vi "FABR-Plot Progress Bars.vi"(0 "Analysis":T1, 2 "Neural Ref":refnum<vi>, 7 "finished":bool, 11 "error in (no error)":errorcluster) -> (15 "error out":errorcluster)   [LabVIEW 2020]
uses:
  Typedefs/FABR-Analysis State.ctl
  Threshold Estimation VIs/ABR3-Threshold Estimation Result.ctl
panel:
  # "Freq X Level X Time"
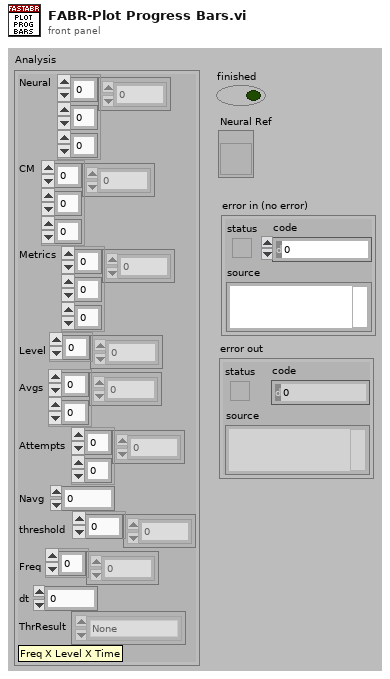
[diagram p1: front panel]
types:
  T1 = typedef "FABR-Analysis State.ctl" = cluster{"Neural":dbl[][][], "CM":dbl[][][], "Metrics":dbl[][][], "Level":dbl[], "Avgs":i32[][], "Attempts":i32[][], "Navg":i32, "threshold":dbl[], "Freq":dbl[], "dt":dbl, "ThrResult":T2[]}
  T2 = typedef "ABR3-Threshold Estimation Result.ctl" = enum16{"None", "Power", "Sigmoid", "Power (noisy)", "Suprathreshold", "Invalid"}
  T3 = typedef "LVRectTypeDef.ctl" = cluster{"Left":i16, "Top":i16, "Right":i16, "Bottom":i16}
  T4 = cluster{"Width":i16, "Style":enum32{"Solid", "Dash", "Dot", "DashDot", "DashDotDot"}}
  T5 = typedef "LVPoint32TypeDef.ctl" = cluster{"Horizontal":i32, "Vertical":i32}
  T6 = cluster{"Horizontal":i32, i32, "Horizontal":i32, i32}
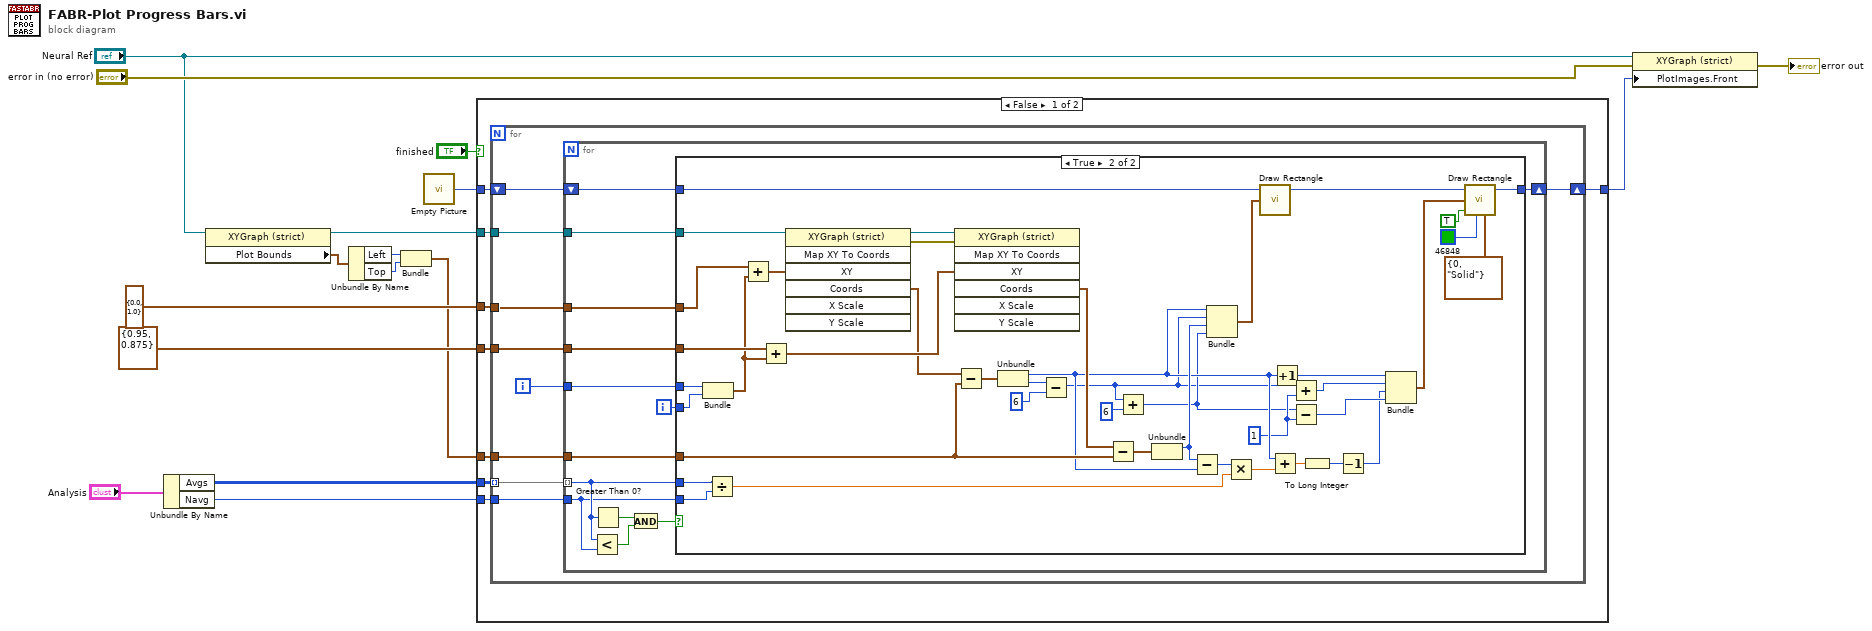
[diagram p0: block diagram]
diagram:
  n1 = Unbundle By Name("Analysis") -> ("Avgs"=w13:i32[][], "Navg"=w8:i32)
  n2 = property class="XYGraph (strict)"(reference="Neural Ref") -> (reference out=w7:refnum<vi>, "Plot Bounds"=w5:T3)  [unwired: 1 in, 1 out]
  n3 = Unbundle By Name(w5) -> ("Left"=w4:i16, "Top"=w3:i16)
  n4 = Bundle("Left"=w4, "Top"=w3) -> (w2:cluster{"Left":i16, "Top":i16})  [unwired: 1 in]
  n5 = call "Empty Picture"() -> ("empty picture"=w12:picture)
  n6 = case shown="False" "finished" {
    tunnel: w13 -> [w24 _]
    tunnel: w12 -> [w23 w90]
    tunnel: [w22 w90] -> w11
    tunnel: cluster{"X":dbl, "Y":dbl} {"X"=0.0, "Y"=1.0} ("XY") -> [w21 _]
    tunnel: cluster{"X":dbl, "Y":dbl} {"X"=0.95, "Y"=0.875} ("XY") -> [w20 _]
    tunnel: w8 -> [w19 _]
    tunnel: w7 -> [w18 _]
    tunnel: w2 -> [w17 _]
    frame False {
      n7 = for {
        tunnel: w24 -> [w28] mode=indexing
        shift-right: [w32] -> w22
        shift-left: w23 -> [w33]
        tunnel: w21 -> [w31]
        tunnel: w18 -> [w29]
        tunnel: w20 -> [w27]
        tunnel: w19 -> [w26]
        tunnel: w17 -> [w25]
        i -> [w30]
        n8 = for {
          shift-right: [w39] -> w32
          shift-left: w33 -> [w46]
          tunnel: w31 -> [w45]
          tunnel: w30 -> [w44]
          tunnel: w29 -> [w42]
          tunnel: w28 -> [w35] mode=indexing
          tunnel: w27 -> [w41]
          tunnel: w26 -> [w34]
          tunnel: w25 -> [w40]
          i -> [w43]
          n9 = Less?(x=w35, y=w34) -> (x < y?=w37:bool)
          n10 = Greater Than 0?(x=w35) -> (x > 0?=w38:bool)
          n11 = And(x=w38, y=w37) -> (x .and. y?=w36:bool)
          n12 = case shown="True" w36 {
            tunnel: w46 -> [w47 w89]
            tunnel: w45 -> [_ w88]
            tunnel: w44 -> [_ w87]
            tunnel: w43 -> [_ w86]
            tunnel: w42 -> [_ w84]
            tunnel: w41 -> [_ w81]
            tunnel: w40 -> [_ w74]
            tunnel: [w47 w72] -> w39
            tunnel: w35 -> [_ w53]
            tunnel: w34 -> [_ w52]
            frame False {
            }
            frame True {
              w59 = 1
              n13 = Bundle(w87, w86) -> (w80:cluster{i32, i32})  [unwired: 1 in]
              n14 = Divide(x=w53, y=w52) -> (x/y=w51:dbl)
              n15 = Add(x=w88, y=w80) -> (x+y=w85:cluster{dbl, dbl})
              n16 = Add(x=w81, y=w80) -> (x+y=w79:cluster{dbl, dbl})
              n17 = invoke class="XYGraph (strict)" method="Map XY To Coords"(reference=w84, "XY"=w85) -> (reference out=w83:refnum<vi>, error out=w82:errorcluster, "Coords"=w78:T5)  [unwired: 5 in, 4 out]
              n18 = invoke class="XYGraph (strict)" method="Map XY To Coords"(reference=w83, error in=w82, "XY"=w79) -> ("Coords"=w77:T5)  [unwired: 4 in, 6 out]
              n19 = Subtract(x=w78, y=w74) -> (x-y=w76:T5)
              n20 = Unbundle(w76) -> ("Horizontal"=w61:i32, "Vertical"=w58:i32)
              n21 = Subtract(x=w58, y=6) -> (x-y=w55:i32)
              n22 = Subtract(x=w77, y=w74) -> (x-y=w75:T5)
              n23 = Add(x=w55, y=6 ("Vertical")) -> (x+y=w56:i32)
              n24 = Unbundle(w75) -> ("Horizontal"=w69:i32)  [unwired: 1 out]
              n25 = Subtract(x=w69, y=w61) -> (x-y=w68:i32)
              n26 = Bundle("Horizontal"=w61, w55, "Horizontal"=w69, w56) -> (w67:T6)  [unwired: 1 in]
              n27 = Multiply(x=w68, y=w51) -> (x*y=w66:dbl)
              n28 = call <vilib>:"Draw Rectangle.vi"("picture"=w89, "rect"=w67) -> ("new picture"=w73:picture)  [unwired: 7 in]
              n29 = Add(x=w61, y=w66) -> (x+y=w64:dbl)
              n30 = Increment(x=w61) -> (x+1=w50:i32)
              n31 = Add(x=w55, y=w59) -> (x+y=w65:i32)
              n32 = Subtract(x=w56, y=w59) -> (x-y=w63:i32)
              n33 = To Long Integer(number=w64) -> (32bit integer=w49:i32)
              n34 = Decrement(x=w49) -> (x-1=w48:i32)
              n35 = Bundle(w50, w65, w48, w63) -> (w62:cluster{i32, i32, i32, i32})  [unwired: 1 in]
              n36 = call <vilib>:"Draw Rectangle.vi"("picture"=w73, "rect"=w62, "fill?(F)"=TRUE, "color(black)"=u32 46848, "pen"=T4 {"Width"=0, "Style"=enum."Solid"}) -> ("new picture"=w72:picture)  [unwired: 4 in]
            }
          }
        }
      }
    }
    frame True {
    }
  }
  n37 = property class="XYGraph (strict)"(reference="Neural Ref", error in="error in (no error)", "PlotImages.Front"=w11) -> (error out=→"error out":errorcluster)  [unwired: 1 out]
